vi "Get Wfm Data Refs.vi"(8 "error in":errorcluster, 11 "State Vars":T2 {"CompiledSettings"."Result Ch Data Refs" format="%.0x"; "CompiledSettings"."Parameter Block Data Refs"."Data Reference" format="%.0x"}) -> (0 "error out":errorcluster, 2 "Source Wfm Data Refs":T1[](array[typedef]), 3 "Result Wfm Data Refs":T1[](array[typedef]))   [LabVIEW 2017, in "Waveform-Processing-Custom-Device Engine.lvlib"]
uses:
  Waveform-Processing-Custom-Device Engine.lvlib
  Types/Inline State Vars.ctl
  Types/Async FIFOs.ctl
  Shared/CompiledSettings.ctl
  <vilib>/NI Veristand/Custom Device API/Block Data Reference.ctl
  <vilib>/NI Veristand/Custom Device API/Data Reference.ctl
  <vilib>/NI Veristand/Custom Device API/Waveform Data Reference.ctl
  <vilib>/NI VeriStand/Custom Device API/Custom Device API.lvlib
  Shared/Waveform-Processing-Custom-Device Shared.lvlib
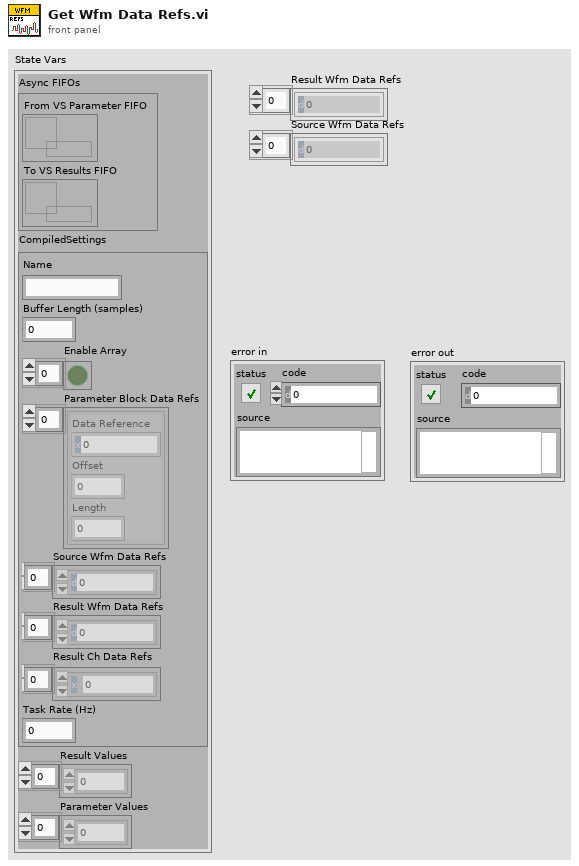
[diagram p1: front panel]
types:
  T1 = typedef "Custom Device API.lvlib/Waveform Data Reference.ctl" = i32
  T2 = typedef "Waveform-Processing-Custom-Device Engine.lvlib/Inline State Vars.ctl" = cluster{"Async FIFOs":T3, "CompiledSettings":T4, "Result Values":dbl[], "Parameter Values":dbl[]}
  T3 = typedef "Waveform-Processing-Custom-Device Engine.lvlib/Async FIFOs.ctl" = cluster{"From VS Parameter FIFO":refnum<k33>, "To VS Results FIFO":refnum<k33>}
  T4 = typedef "Waveform-Processing-Custom-Device Shared.lvlib/CompiledSettings.ctl" = cluster{"Name":string, "Buffer Length (samples)":u32, "Enable Array":bool[], "Parameter Block Data Refs":T5[], "Source Wfm Data Refs":T1[], "Result Wfm Data Refs":T1[], "Result Ch Data Refs":T6[], "Task Rate (Hz)":dbl}
  T5 = typedef "Custom Device API.lvlib/Block Data Reference.ctl" = cluster{"Data Reference":T6, "Offset":u64, "Length":u64}
  T6 = typedef "Custom Device API.lvlib/Data Reference.ctl" = i32
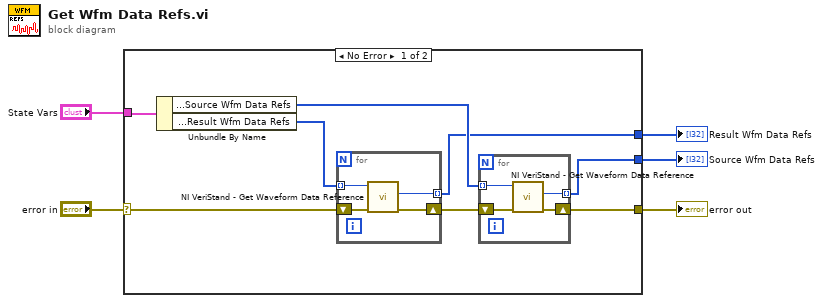
[diagram p0: block diagram]
diagram:
  n1 = case shown="No Error" "error in" {
    selector: "error in" -> [w12 w22]
    tunnel: "State Vars" -> [w13 _]
    tunnel: [w8 _] -> w2
    tunnel: [w7 _] -> w1
    tunnel: [w6 w22] -> w3
    frame No Error {
      n2 = Unbundle By Name(w13) -> ("CompiledSettings.Source Wfm Data Refs"=w9:T1[], "CompiledSettings.Result Wfm Data Refs"=w11:T1[])
      n3 = for {
        tunnel: w11 -> [w20] mode=indexing
        tunnel: [w18] -> w8 mode=indexing
        shift-right: [w19] -> w10
        shift-left: w12 -> [w21]
        n4 = call <vilib>:"NI VeriStand - Get Waveform Data Reference.vi"("error in (no error)"=w21, "Waveform Ref in"=w20) -> ("error out"=w19:errorcluster, "Waveform Data Reference"=w18:T1)  [unwired: 7 in, 1 out]
      }
      n5 = for {
        tunnel: w9 -> [w16] mode=indexing
        tunnel: [w15] -> w7 mode=indexing
        shift-right: [w14] -> w6
        shift-left: w10 -> [w17]
        n6 = call <vilib>:"NI VeriStand - Get Waveform Data Reference.vi"("error in (no error)"=w17, "Waveform Ref in"=w16) -> ("error out"=w14:errorcluster, "Waveform Data Reference"=w15:T1)  [unwired: 7 in, 1 out]
      }
    }
    frame Error {
    }
  }
  "error out" <- w3
  "Result Wfm Data Refs" <- w2
  "Source Wfm Data Refs" <- w1
